vi "Decode Spreadsheet String to 2D Array.vi"(6 "Delimiter (,)":string=",", 8 "error in (no error)":errorcluster, 11 "Spreadsheet String":string) -> (0 "error out":errorcluster, 3 "2D Array":string[][](array[string]))   [LabVIEW 2016, in "SLL Spreadsheet.lvlib"]
doc: "This converts a Spreadsheet String to a 2D String array even when an individual cell contains characters which are not supported by the built-in Spreadsheet String to Array function (like new line characters)."
uses:
  SLL Spreadsheet.lvlib
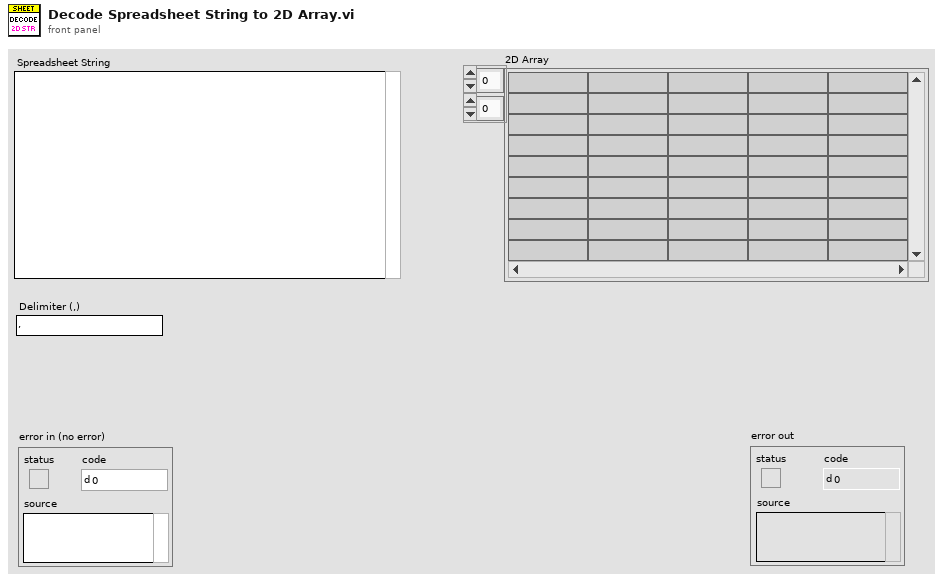
[diagram p1: front panel]
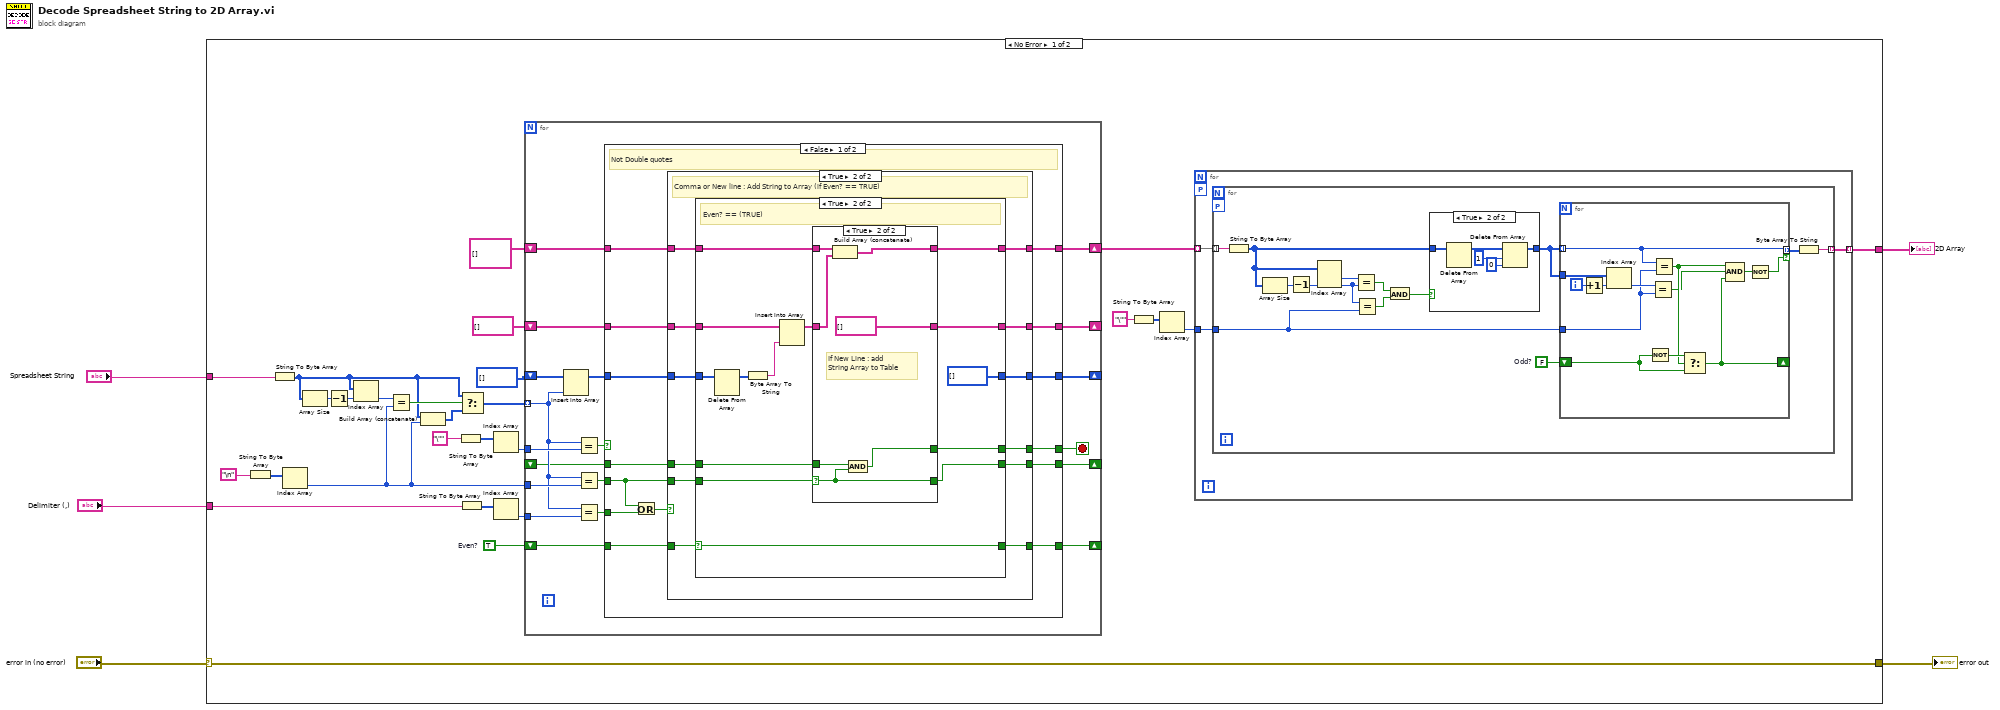
[diagram p0: block diagram]
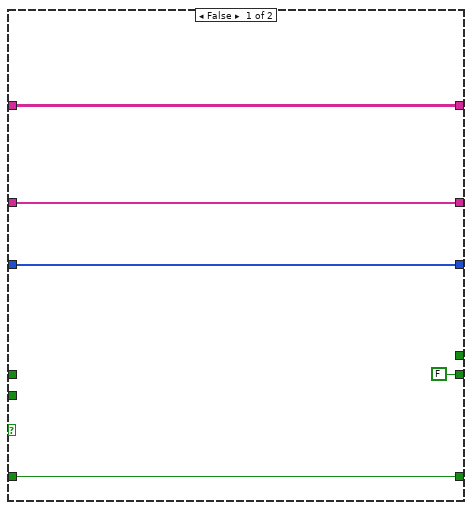
[diagram p3: hidden frame]
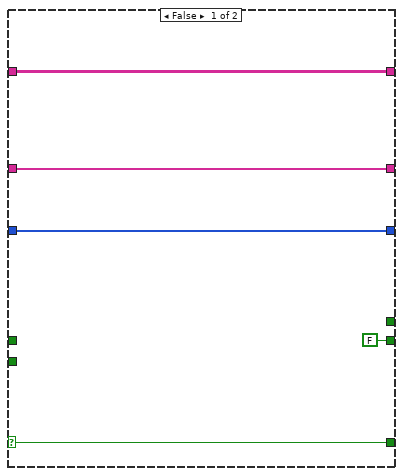
[diagram p4: hidden frame]
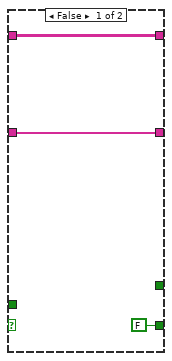
[diagram p5: hidden frame]
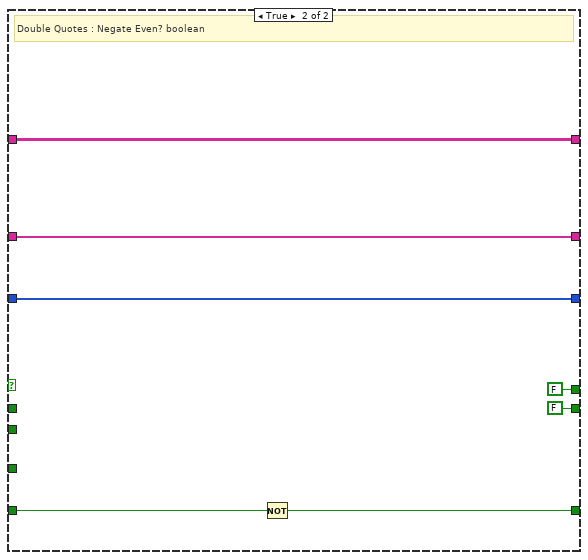
[diagram p6: hidden frame]
diagram:
  n1 = case shown="No Error" "error in (no error)" {
    selector: "error in (no error)" -> [w6 w155]
    tunnel: "Delimiter (,)" -> [w30 _]
    tunnel: [w19 _] -> w4
    tunnel: "Spreadsheet String" -> [w15 _]
    tunnel: [w6 w155] -> w1
    frame No Error {
      w24 = TRUE  # Even?
      n2 = String To Byte Array(string="\n") -> (unsigned byte array=w28:u8[])
      n3 = String To Byte Array(string=w15) -> (unsigned byte array=w8:u8[])
      n4 = Index Array(array=w28) -> (element=w7:u8)  [unwired: 1 in]
      n5 = Array Size(array=w8) -> (size(s)=w14:i32)
      n6 = Decrement(x=w14) -> (x-1=w13:i32)
      n7 = Index Array(array=w8, index=w13) -> (element=w12:u8)
      n8 = Equal?(x=w12, y=w7) -> (x = y?=w11:bool)
      n9 = Build Array (concatenate)(w8, w7) -> (w9:u8[])
      n10 = String To Byte Array(string="\"") -> (unsigned byte array=w29:u8[])
      n11 = String To Byte Array(string=w30) -> (unsigned byte array=w27:u8[])
      n12 = Select(t=w8, s=w11, f=w9) -> (s? t:f=w10:u8[])
      n13 = Index Array(array=w29) -> (element=w26:u8)  [unwired: 1 in]
      n14 = Index Array(array=w27) -> (element=w25:u8)  [unwired: 1 in]
      n15 = for {
        tunnel: w10 -> [w72] mode=indexing
        tunnel: w26 -> [w75]
        tunnel: w7 -> [w74]
        tunnel: w25 -> [w73]
        shift-right: [w83] -> _
        shift-left: w24 -> [w84]
        shift-right: [w81] -> _
        shift-left: u8[] [] -> [w80]
        shift-right: [w78] -> _
        shift-left: string[] [] -> [w79]
        shift-right: [w76] -> w32
        shift-left: string[][] [] -> [w77]
        shift-right: [w71] -> _
        shift-left: _ -> [w70]
        stop <- w69 stop-if-true
        n16 = Insert Into Array(array=w80, new element=w72) -> (w82:u8[])  [unwired: 1 in]
        n17 = Equal?(x=w72, y=w75) -> (x = y?=w87:bool)
        n18 = Equal?(x=w72, y=w74) -> (x = y?=w86:bool)
        n19 = Equal?(x=w72, y=w73) -> (x = y?=w85:bool)
        n20 = case shown="False" w87 {
          tunnel: w86 -> [w91 _]
          tunnel: w85 -> [w92 _]
          tunnel: w84 -> [w101 w154]
          tunnel: [w100 w153] -> w83
          tunnel: w82 -> [w99 w150]
          tunnel: [w98 w150] -> w81
          tunnel: w79 -> [w97 w152]
          tunnel: [w96 w152] -> w78
          tunnel: w77 -> [w95 w151]
          tunnel: [w94 w151] -> w76
          tunnel: [w90 FALSE] -> w71
          tunnel: w70 -> [w89 _]
          tunnel: [w88 FALSE] -> w69
          frame False {
            # "Not Double quotes"
            n21 = Or(x=w91, y=w92) -> (x .or. y?=w93:bool)
            n22 = case shown="True" w93 {
              tunnel: w101 -> [w105 w118]
              tunnel: [w105 w113] -> w100
              tunnel: w99 -> [w104 w115]
              tunnel: [w104 w114] -> w98
              tunnel: w97 -> [w103 w117]
              tunnel: [w103 w116] -> w96
              tunnel: w95 -> [w106 w112]
              tunnel: [w106 w111] -> w94
              tunnel: w91 -> [_ w110]
              tunnel: [FALSE w109] -> w90
              tunnel: w89 -> [_ w108]
              tunnel: [_ w107] -> w88
              frame False {
              }
              frame True {
                # "Comma or New line : Add String to Array (if Even? == TRUE)"
                n23 = case shown="True" w118 {
                  selector: w118 -> [w121 w137]
                  tunnel: [w123 w134] -> w116
                  tunnel: w117 -> [w123 w132]
                  tunnel: [w122 u8[] []] -> w114
                  tunnel: w115 -> [w122 w128]
                  tunnel: [w121 w137] -> w113
                  tunnel: w112 -> [w120 w136]
                  tunnel: [w120 w133] -> w111
                  tunnel: w110 -> [_ w127]
                  tunnel: [FALSE w126] -> w109
                  tunnel: w108 -> [_ w125]
                  tunnel: [_ w124] -> w107
                  frame False {
                  }
                  frame True {
                    # "Even? == (TRUE)"
                    n24 = Delete From Array(array=w128) -> (array with subset deleted=w129:u8[])  [unwired: 2 in, 1 out]
                    n25 = Byte Array To String(unsigned byte array=w129) -> (string=w130:string)
                    n26 = Insert Into Array(array=w132, new element=w130) -> (w131:string[])  [unwired: 1 in]
                    n27 = case shown="True" w127 {
                      selector: w127 -> [_ w142]
                      tunnel: w136 -> [w140 w147]
                      tunnel: [w139 string[] []] -> w134
                      tunnel: [w140 w145] -> w133
                      tunnel: w131 -> [w139 w144]
                      tunnel: [FALSE w142] -> w126
                      tunnel: w125 -> [_ w143]
                      tunnel: [_ w141] -> w124
                      frame False {
                      }
                      frame True {
                        # "If New Line : add String Array to Table"
                        n28 = Build Array (concatenate)(w147, w144) -> (w145:string[][])
                        n29 = And(x=w143, y=w142) -> (x .and. y?=w141:bool)
                      }
                    }
                  }
                }
              }
            }
          }
          frame True {
            # "Double Quotes : Negate Even? boolean"
            n30 = Not(x=w154) -> (.not. x?=w153:bool)
          }
        }
      }
      n31 = String To Byte Array(string="\"") -> (unsigned byte array=w17:u8[])
      n32 = Index Array(array=w17) -> (element=w16:u8)  [unwired: 1 in]
      n33 = for {
        tunnel: w32 -> [w35] mode=indexing
        tunnel: w16 -> [w34]
        tunnel: [w33] -> w19 mode=indexing
        workers-P: _ -> [_]
        n34 = for {
          tunnel: w35 -> [w49] mode=indexing
          tunnel: w34 -> [w39]
          tunnel: [w37] -> w33 mode=indexing
          workers-P: _ -> [_]
          w36 = FALSE  # Odd?
          n35 = String To Byte Array(string=w49) -> (unsigned byte array=w41:u8[])
          n36 = Array Size(array=w41) -> (size(s)=w48:i32)
          n37 = Decrement(x=w48) -> (x-1=w47:i32)
          n38 = Index Array(array=w41, index #2=w47) -> (element #1=w46:u8, element #2=w45:u8)  [unwired: 1 in]
          n39 = Equal?(x=w46, y=w45) -> (x = y?=w43:bool)
          n40 = Equal?(x=w45, y=w39) -> (x = y?=w44:bool)
          n41 = And(x=w43, y=w44) -> (x .and. y?=w42:bool)
          n42 = case shown="True" w42 {
            tunnel: w41 -> [w63 w68]
            tunnel: [w63 w66] -> w40
            frame False {
            }
            frame True {
              n43 = Delete From Array(array=w68) -> (array with subset deleted=w67:u8[])  [unwired: 2 in, 1 out]
              n44 = Delete From Array(array=w67, length=1, index=0) -> (array with subset deleted=w66:u8[])  [unwired: 1 out]
            }
          }
          n45 = for {
            tunnel: w40 -> [w57] mode=indexing
            tunnel: w40 -> [w62]
            tunnel: w39 -> [w58]
            tunnel: [w57] -> w38 mode=indexing if=w56
            shift-right: [w51] -> _
            shift-left: w36 -> [w55]
            i -> [w61]
            n46 = Increment(x=w61) -> (x+1=w60:i32)
            n47 = Index Array(array=w62, index=w60) -> (element=w59:u8)
            n48 = Not(x=w55) -> (.not. x?=w54:bool)
            n49 = Equal?(x=w59, y=w58) -> (x = y?=w52:bool)
            n50 = Equal?(x=w57, y=w58) -> (x = y?=w53:bool)
            n51 = Select(t=w54, s=w53, f=w55) -> (s? t:f=w51:bool)
            n52 = Compound Arithmetic op=AND(w53, w52, w51) -> (w50:bool)
            n53 = Not(x=w50) -> (.not. x?=w56:bool)
          }
          n54 = Byte Array To String(unsigned byte array=w38) -> (string=w37:string)
        }
      }
    }
    frame Error {
    }
  }
  "2D Array" <- w4
  "error out" <- w1
